vi "ep_Evaluate Digital Formula.vi"(0 "digital formula":string, 5 "digital variables":bool[](array[boolean]), 11 "error in (no error)":errorcluster) -> (4 "result":bool, 15 "error out":errorcluster)   [LabVIEW 2011, in "NI_EP_Power Quality.lvlib"]
uses:
  <vilib>/addons/Electrical Power/PQ/NI_EP_Power Quality.lvlib
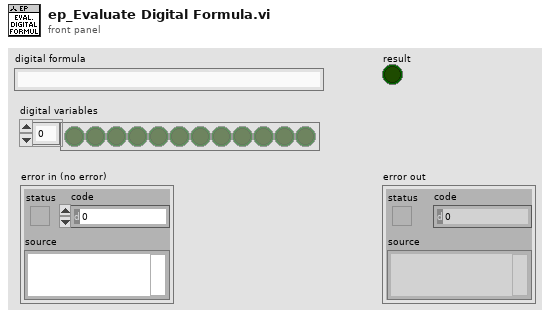
[diagram p1: front panel]
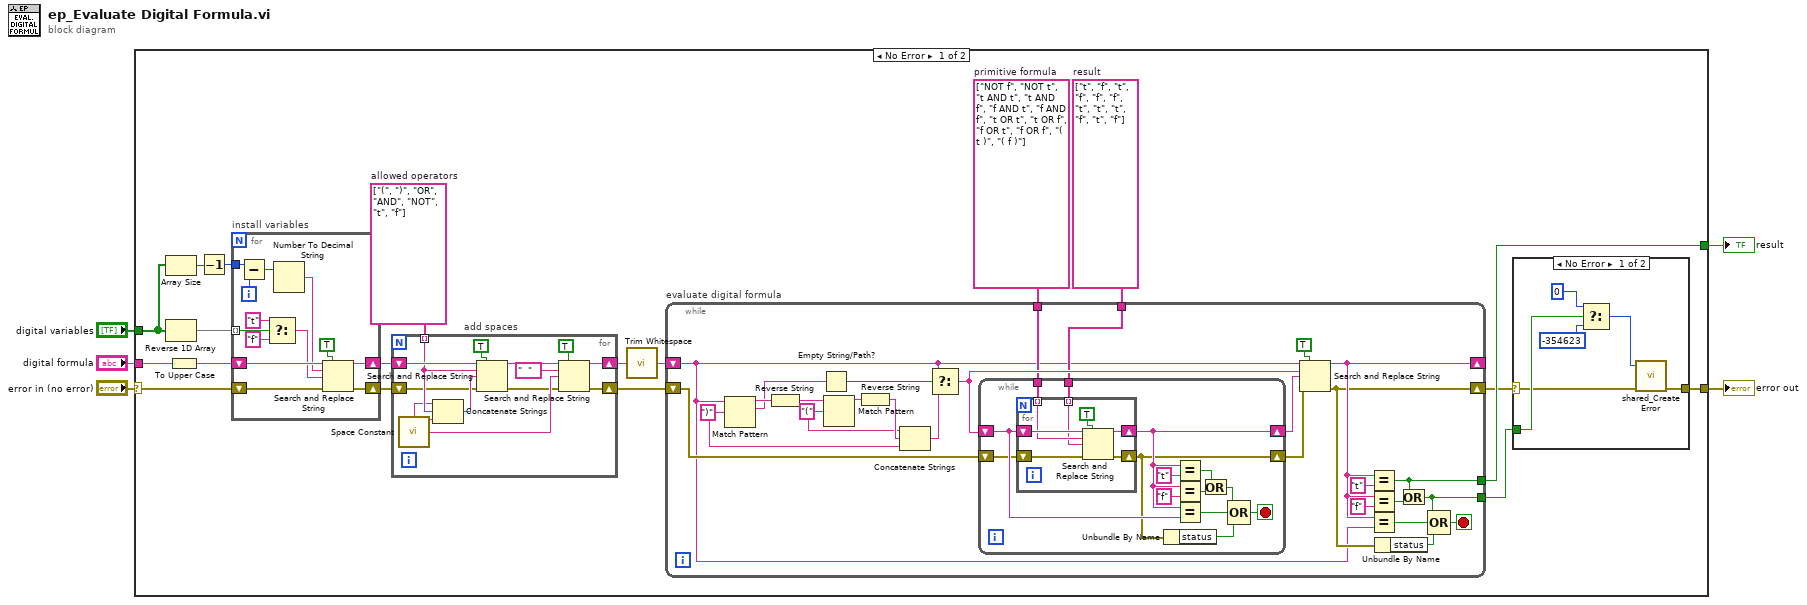
[diagram p0: block diagram]
diagram:
  n1 = case shown="No Error" "error in (no error)" {
    selector: "error in (no error)" -> [w13 w105]
    tunnel: "digital variables" -> [w19 _]
    tunnel: [w8 _] -> w4
    tunnel: "digital formula" -> [w17 _]
    tunnel: [w14 w105] -> w2
    frame No Error {
      w11 = string[] ["t", "f", "t", "f", "f", "f", "t", "t", "t", "f", "t", "f"]  # result
      w12 = string[] ["NOT f", "NOT t", "t AND t", "t AND f", "f AND t", "f AND f", "t OR t", "t OR f", "f OR t", "f OR f", "( t )", "( f )"]  # primitive formula
      w21 = string[] ["(", ")", "OR", "AND", "NOT", "t", "f"]  # allowed operators
      n2 = Array Size(array=w19) -> (size(s)=w23:i32)
      n3 = Reverse 1D Array(array=w19) -> (reversed array=w24:bool[])
      n4 = To Upper Case(1:w17) -> (0:w16:string)
      n5 = Decrement(x=w23) -> (x-1=w22:i32)
      n6 = for "install variables" {
        tunnel: w24 -> [w100] mode=indexing
        shift-right: [w94] -> w18
        shift-left: w16 -> [w104]
        tunnel: w22 -> [w103]
        shift-right: [w95] -> w15
        shift-left: w13 -> [w96]
        i -> [w102]
        n7 = Subtract(x=w103, y=w102) -> (x-y=w101:i32)
        n8 = Select(t="t", s=w100, f="f") -> (s? t:f=w97:string)
        n9 = Number To Decimal String(number=w101) -> (decimal integer string=w92:string)  [unwired: 1 in]
        n10 = Search and Replace String(replace all?=TRUE ("replace all? (F)"), input string=w104, search string=w92, replace string=w97, error in=w96) -> (result string=w94:string, error out=w95:errorcluster)  [unwired: 3 in, 2 out]
      }
      n11 = for "add spaces" {
        tunnel: w21 -> [w84] mode=indexing
        shift-right: [w86] -> w20
        shift-left: w18 -> [w90]
        shift-right: [w80] -> w9
        shift-left: w15 -> [w82]
        n12 = call <vilib>:"Space Constant.vi"() -> ("String"=w83:string)
        n13 = Concatenate Strings(w83, w84, w83) -> (w85:string)
        n14 = Search and Replace String(replace all?=TRUE ("replace all? (F)"), input string=w90, search string=w84, replace string=w85, error in=w82) -> (result string=w87:string, error out=w81:errorcluster)  [unwired: 3 in, 2 out]
        n15 = Search and Replace String(replace all?=TRUE ("replace all? (F)"), input string=w87, search string="  ", replace string=w83, error in=w81) -> (result string=w86:string, error out=w80:errorcluster)  [unwired: 3 in, 2 out]
      }
      n16 = call <vilib>:"Trim Whitespace.vi"("string"=w20) -> ("trimmed string"=w10:string)  [unwired: 1 in]
      n17 = while "evaluate digital formula" {
        shift-right: [w39] -> _
        shift-left: w10 -> [w27]
        shift-right: [w31] -> w7
        shift-left: w9 -> [w32]
        tunnel: w12 -> [w29]
        tunnel: w11 -> [w28]
        tunnel: [w26] -> w8
        tunnel: [w25] -> w6
        stop <- w40 stop-if-true
        w47 = "(" ("regular expression")
        w46 = ")" ("regular expression")
        n18 = Match Pattern(string=w27, regular expression=w46) -> (before substring=w51:string, match substring=w38:string)  [unwired: 1 in, 2 out]
        n19 = Reverse String(1:w51) -> (0:w50:string)
        n20 = Empty String/Path?(string/path=w38) -> (empty?=w37:bool)
        n21 = Match Pattern(string=w50, regular expression=w47) -> (before substring=w49:string)  [unwired: 1 in, 3 out]
        n22 = Reverse String(1:w49) -> (0:w48:string)
        n23 = Concatenate Strings(w47, w48, w46) -> (w36:string)
        n24 = Select(t=w27, s=w37, f=w36) -> (s? t:f=w35:string)
        n25 = while {
          shift-right: [w54] -> w34
          shift-left: w35 -> [w62]
          shift-right: [w53] -> w33
          shift-left: w32 -> [w57]
          tunnel: w29 -> [w56]
          tunnel: w28 -> [w55]
          stop <- w59 stop-if-true
          n26 = for {
            shift-right: [w70] -> w54
            shift-left: w62 -> [w71]
            tunnel: w56 -> [w69] mode=indexing
            tunnel: w55 -> [w68] mode=indexing
            shift-right: [w66] -> w53
            shift-left: w57 -> [w67]
            n27 = Search and Replace String(replace all?=TRUE ("replace all? (F)"), input string=w71, search string=w69, replace string=w68, error in=w67) -> (result string=w70:string, error out=w66:errorcluster)  [unwired: 3 in, 2 out]
          }
          n28 = Unbundle By Name(w53) -> ("status"=w52:bool)
          n29 = Equal?(x=w54, y="t") -> (x = y?=w58:bool)
          n30 = Equal?(x=w54, y="f") -> (x = y?=w63:bool)
          n31 = Equal?(x=w54, y=w62) -> (x = y?=w61:bool)
          n32 = Or(x=w58, y=w63) -> (x .or. y?=w60:bool)
          n33 = Compound Arithmetic op=OR(w60, w61, w52) -> (w59:bool)
        }
        n34 = Search and Replace String(replace all?=TRUE ("replace all? (F)"), input string=w27, search string=w35, replace string=w34, error in=w33) -> (result string=w39:string, error out=w31:errorcluster)  [unwired: 3 in, 2 out]
        n35 = Equal?(x=w39, y="t") -> (x = y?=w26:bool)
        n36 = Equal?(x=w39, y="f") -> (x = y?=w43:bool)
        n37 = Equal?(x=w39, y=w27) -> (x = y?=w44:bool)
        n38 = Unbundle By Name(w31) -> ("status"=w30:bool)
        n39 = Or(x=w26, y=w43) -> (x .or. y?=w25:bool)
        n40 = Compound Arithmetic op=OR(w25, w44, w30) -> (w40:bool)
      }
      n41 = case shown="No Error" w7 {
        selector: w7 -> [w75 w79]
        tunnel: w6 -> [w78 _]
        tunnel: [w74 w79] -> w14
        frame No Error {
          n42 = Select(t=0 ("error code (0)"), s=w78, f=-354623 ("error code (0)")) -> (s? t:f=w73:i32)
          n43 = call <vilib>:"shared_Create Error.vi"("error in (no error)"=w75, "error code (0)"=w73) -> ("error out"=w74:errorcluster)  [unwired: 9 in]
        }
        frame Error {
        }
      }
    }
    frame Error {
    }
  }
  "result" <- w4
  "error out" <- w2
